vi "csv-log-data.vi"(0 "log file Byte Stream File in":refnum<file>, 1 "log file path":path, 2 "Datalogging options":T1={"data-precision"=3, "Include Date"=FALSE, "Include Timestamp"=TRUE, "Include Milliseconds"=FALSE}, 5 "Data Array In":dbl[](array[numeric]), 7 "Data Point In":dbl, 9 "File Open?":bool=TRUE, 11 "error in (no error)":errorcluster, 13 "Override Format Array?":bool, 14 "Format Array Override":string="%.2f") -> (3 "log file path":path, 4 "log file Byte Stream File out":refnum<file>, 6 "time string":string, 8 "Logged CSV out":string, 15 "error out":errorcluster)   [LabVIEW 2024]
uses:
  datalogging-options.ctl
panel:
  out "format array to string":string="%.2f"
  out "datapoints string":string
  # "If \"File Open\" byte stream is used\nelse File Path is used"
  # "Current Timestamp for Logging"
  # "If overriding format array \"Format Array Override\"\nmust have valid format string (%.2f) for float with \n2 digit precision after decimal point"
  # "This is the string that will be logged to file"
  # "The format string used \nto format array data to \ndatapoints string"
  # "The formated string created from Data Array In"
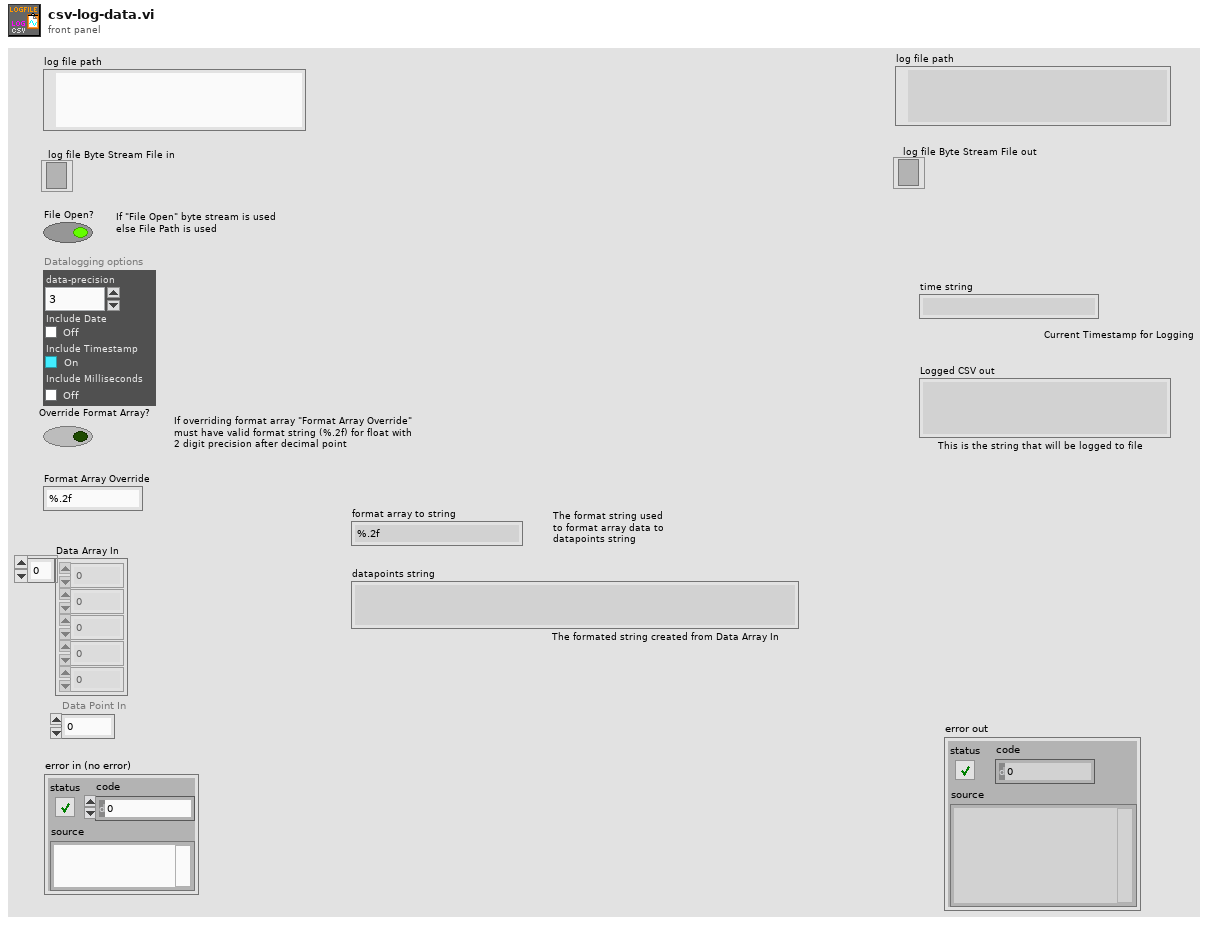
[diagram p1: front panel]
types:
  T1 = typedef "datalogging-options.ctl" = cluster{"data-precision":i32, "Include Date":bool, "Include Timestamp":bool, "Include Milliseconds":bool}
  T2 = enum16{"open", "replace", "create", "open or create", "replace or create", "replace or create with confirmation"}
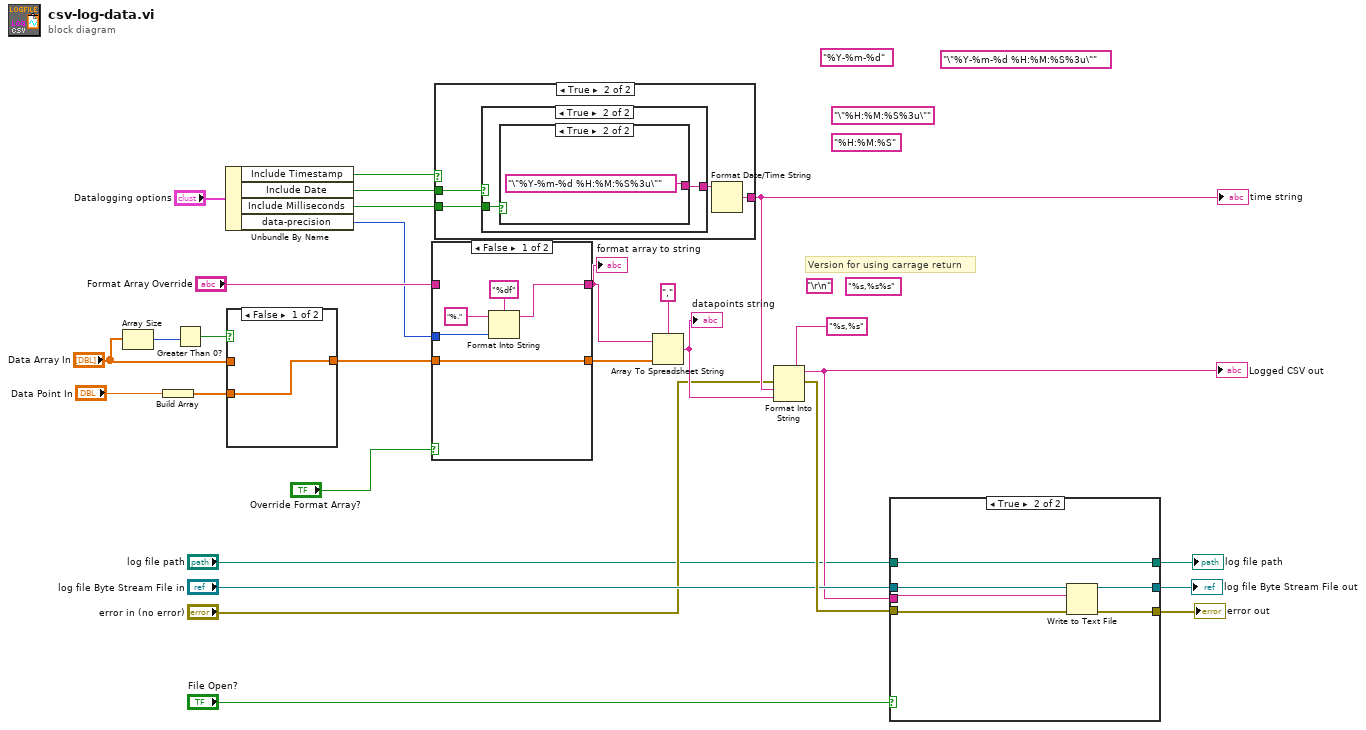
[diagram p0: block diagram]
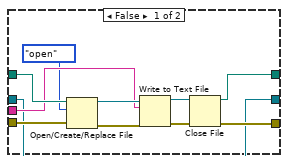
[diagram p4: hidden frame]
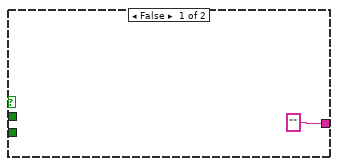
[diagram p5: hidden frame]
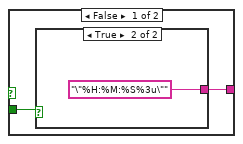
[diagram p6: hidden frame]
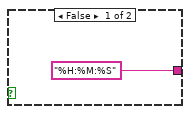
[diagram p7: hidden frame]
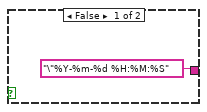
[diagram p8: hidden frame]
diagram:
  (unwired) "%Y-%m-%d" ("time format string (%c)")
  (unwired) "\"%Y-%m-%d %H:%M:%S%3u\"" ("time format string (%c)")
  (unwired) "%H:%M:%S" ("time format string (%c)")
  (unwired) "\"%H:%M:%S%3u\"" ("time format string (%c)")
  (unwired) "%s,%s%s" ("format string")
  (unwired) "\r\n"
  # "Version for using carrage return"
  n1 = Array Size(array="Data Array In") -> (size(s)=w9:i32)
  n2 = Build Array("Data Point In") -> (w5:dbl[])
  n3 = Greater Than 0?(x=w9) -> (x > 0?=w7:bool)
  n4 = Unbundle By Name("Datalogging options") -> ("Include Timestamp"=w28:bool, "Include Date"=w1:bool, "Include Milliseconds"=w2:bool, "data-precision"=w3:i32)
  n5 = case shown="False" w7 {
    tunnel: [w29 w30] -> w6
    tunnel: w5 -> [w29 _]
    tunnel: "Data Array In" -> [_ w30]
    frame False {
    }
    frame True {
    }
  }
  n6 = case shown="False" "Override Format Array?" {
    tunnel: w3 -> [w33 _]
    tunnel: [w32 w37] -> w11
    tunnel: "Format Array Override" -> [_ w37]
    tunnel: [w31 w36] -> w10
    tunnel: w6 -> [w31 w36]
    frame False {
      n7 = Format Into String "Format Into String"(format string="%df", initial string="%.", w33) -> (resulting string=w32:string)  [unwired: 1 in, 1 out]
    }
    frame True {
    }
  }
  "format array to string" <- w11
  n8 = case shown="True" w28 {
    tunnel: ["" ("date/time string") w42] -> w26
    tunnel: w2 -> [_ w40]
    tunnel: w1 -> [_ w39]
    frame False {
    }
    frame True {
      n9 = case shown="True" w39 {
        tunnel: [w44 w48] -> w41
        tunnel: w40 -> [w43 w47]
        frame False {
          n10 = case shown="True" w43 {
            tunnel: ["%H:%M:%S" ("time format string (%c)") "\"%H:%M:%S%3u\"" ("time format string (%c)")] -> w44
            frame False {
            }
            frame True {
            }
          }
        }
        frame True {
          n11 = case shown="True" w47 {
            tunnel: ["\"%Y-%m-%d %H:%M:%S" ("time format string (%c)") "\"%Y-%m-%d %H:%M:%S%3u\"" ("time format string (%c)")] -> w48
            frame False {
            }
            frame True {
            }
          }
        }
      }
      n12 = Format Date/Time String(time format string (%c)=w41) -> (date/time string=w42:string)  [unwired: 2 in]
    }
  }
  "time string" <- w26
  n13 = Array To Spreadsheet String(delimiter (Tab)=",", array=w10, 3:w11) -> (spreadsheet string=w25:string)
  "datapoints string" <- w25
  n14 = Format Into String "Format Into String"(format string="%s,%s", error in="error in (no error)", w26, w25) -> (resulting string=w19:string, error out=w21:errorcluster)  [unwired: 1 in]
  "Logged CSV out" <- w19
  n15 = case shown="True" "File Open?" {
    tunnel: [w57 w67] -> w23
    tunnel: [w51 w66] -> w22
    tunnel: w21 -> [w53 w65]
    tunnel: "log file Byte Stream File in" -> [w51 w64]
    tunnel: w19 -> [w54 w63]
    tunnel: "log file path" -> [w55 w62]
    tunnel: [w56 w62] -> w15
    frame False {
      n16 = Open/Create/Replace File(file path (use dialog)=w55, error in=w53, operation (0:open)=T2."open") -> (refnum out=w59:refnum<file>, error out=w58:errorcluster)  [unwired: 3 in, 1 out]
      n17 = Write to Text File(file (use dialog)=w59, text=w54, error in=w58) -> (refnum out=w60:refnum<file>, error out=w61:errorcluster)  [unwired: 1 in, 1 out]
      n18 = Close File(refnum=w60, error in=w61) -> (path=w56:path, error out=w57:errorcluster)
    }
    frame True {
      n19 = Write to Text File(file (use dialog)=w64, text=w63, error in=w65) -> (refnum out=w66:refnum<file>, error out=w67:errorcluster)  [unwired: 1 in, 1 out]
    }
  }
  "error out" <- w23
  "log file Byte Stream File out" <- w22
  "log file path" <- w15
